vi "Assert TimeStamp.vi"() -> ()   [LabVIEW 2015]
uses:
  <vilib>/Utility/miscctls.llb/LVDateTimeRec.ctl
panel:
  out "x-y":T1
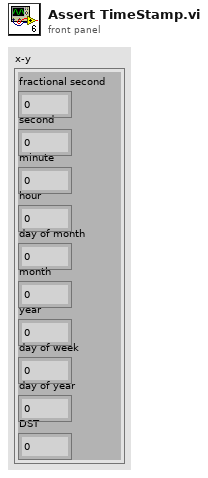
[diagram p1: front panel]
types:
  T1 = typedef "LVDateTimeRec.ctl" = cluster{"fractional second":dbl, "second":i32, "minute":i32, "hour":i32, "day of month":i32, "month":i32, "year":i32, "day of week":i32, "day of year":i32, "DST":i32}
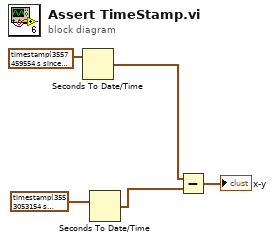
[diagram p0: block diagram]
diagram:
  n1 = Seconds To Date/Time(time stamp (now)=timestamp(3557459554.214689 s since 1904-01-01) ("Time Stamp")) -> (date time rec=w5:T1)  [unwired: 1 in]
  n2 = Seconds To Date/Time(time stamp (now)=timestamp(3553053154.214689 s since 1904-01-01) ("Time Stamp")) -> (date time rec=w3:T1)  [unwired: 1 in]
  n3 = Subtract(x=w5, y=w3) -> (x-y=→"x-y":T1)
